vi "Test_PanelValueInit.vi"(8 "error in (no error)":errorcluster, 11 "Test.Maui 2.0.Panels in":refnum<class "Test.Maui 2.0.Panels.lvclass">) -> (0 "error out":errorcluster, 3 "Test.Maui 2.0.Panels out":refnum<class "Test.Maui 2.0.Panels.lvclass">)   [LabVIEW 2020, in "Test.Maui 2.0.Panels.lvclass"]
uses:
  Test.Maui 2.0.Panels.lvclass
  Test.Maui 2.0.Panels.lvclass/Test.Maui 2.0.Panels.ctl
  <vilib>/addons/_JKI Toolkits/Caraya/classes/Assert/Assert Equal Value_Variant.vi
  <vilib>/addons/_JKI Toolkits/Caraya/classes/Assert/Assert Not Error.vi
  Helper/Test Helper 1/Test Helper 1.lvclass
  <vilib>/addons/_JKI Toolkits/Caraya/classes/Assert/Assert.lvclass
  <vilib>/addons/_JKI Toolkits/Caraya/classes/Test/Test.lvclass
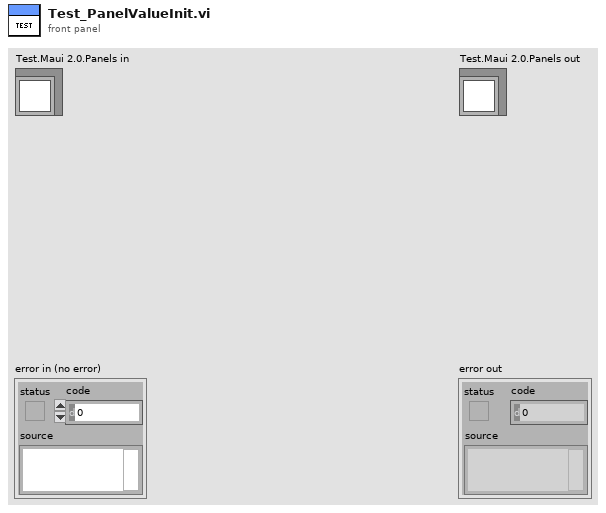
[diagram p1: front panel]
types:
  T1 = cluster{"Ring 2":refnum<vi>, "Sub Panel 2":refnum<vi>}[]
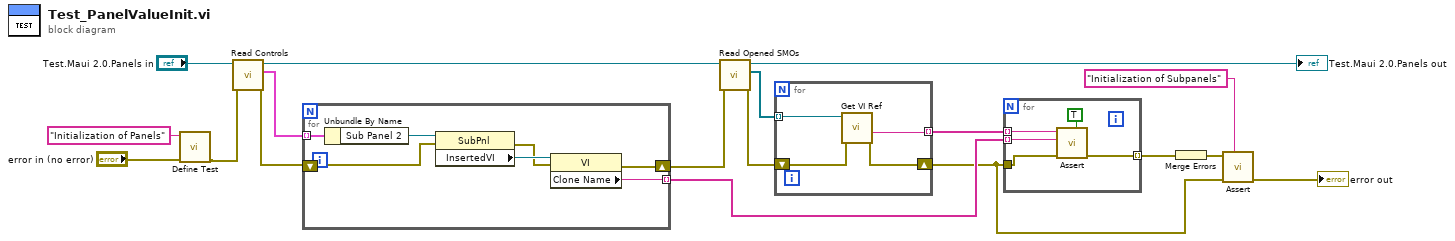
[diagram p0: block diagram]
diagram:
  n1 = call <vilib>:"Define Test.vi"("error in (no error)"="error in (no error)", "Label (VI Title)"="Initialization of Panels") -> ("error out"=w2:errorcluster)  [unwired: 9 in]
  n2 = call "Read Controls.vi"("error in (no error)"=w2, "Test.Maui 2.0.Panels in"="Test.Maui 2.0.Panels in") -> ("error out"=w16:errorcluster, "Controls"=w17:T1, "Test.Maui 2.0.Panels out"=w15:refnum<class "Test.Maui 2.0.Panels.lvclass">)  [unwired: 7 in]
  n3 = for {
    tunnel: w17 -> [w25] mode=indexing
    tunnel: [w22] -> w9 mode=indexing
    shift-right: [w19] -> w13
    shift-left: w16 -> [w20]
    n4 = Unbundle By Name(w25) -> ("Sub Panel 2"=w24:refnum<vi>)
    n5 = property on="Property Node" class="SubPnl"(reference=w24, error in=w20) -> (error out=w21:errorcluster, "InsertedVI"=w23:refnum<vi>)  [unwired: 1 out]
    n6 = property on="Property Node" class="VI"(reference=w23, error in=w21) -> (error out=w19:errorcluster, "Clone Name"=w22:string)  [unwired: 1 out]
  }
  n7 = call "Read Opened SMOs.vi"("error in (no error)"=w13, "Test.Maui 2.0.Panels in"=w15) -> ("error out"=w11:errorcluster, "Opened SMOs"=w12:refnum<class "Test Helper 1.lvclass">[], "Test.Maui 2.0.Panels out"=→"Test.Maui 2.0.Panels out":refnum<class "Test.Maui 2.0.Panels.lvclass">)  [unwired: 7 in]
  n8 = for {
    tunnel: w12 -> [w29] mode=indexing
    shift-right: [w26] -> w6
    shift-left: w11 -> [w27]
    tunnel: [w28] -> w10 mode=indexing
    n9 = call-dynamic "Get VI Ref.vi"("error in (no error)"=w27, "Test Helper 1 in"=w29) -> ("error out"=w26:errorcluster, "VI Clone Name"=w28:string)  [unwired: 6 in, 2 out]
  }
  n10 = for {
    tunnel: w10 -> [w34] mode=indexing
    tunnel: w9 -> [w33] mode=indexing
    tunnel: w6 -> [w32]
    tunnel: [w31] -> w8 mode=indexing
    n11 = call-poly <vilib>:"Assert.vi"("Assert Only? (F)"=TRUE, "error in (no error)"=w32, "Y"=w33, "X"=w34) -> ("error out"=w31:errorcluster)  [unwired: 7 in]
  }
  n12 = Merge Errors(w8) -> (w7:errorcluster)
  n13 = call-poly <vilib>:"Assert.vi"("Label"="Initialization of Subpanels", "error in (no error)"=w6, "Not Error?"=w7) -> ("error out"=→"error out":errorcluster)  [unwired: 8 in]
